vi "CalculateFit.vi"(8 "error in (no error)":errorcluster, 9 "Response in":dbl[][](array[numeric]), 10 "Stimulus in":dbl[][](array[numeric]), 11 "Head Impulse Fit in":refnum<class "Head Impulse Fit.lvclass">) -> (0 "error out":errorcluster, 3 "Head Impulse Fit out":refnum<class "Head Impulse Fit.lvclass">)   [LabVIEW 2016, in "Head Impulse Fit.lvclass"]
uses:
  Head Impulse Fit.lvclass
  Head Impulse Fit.lvclass/Head Impulse Fit.ctl
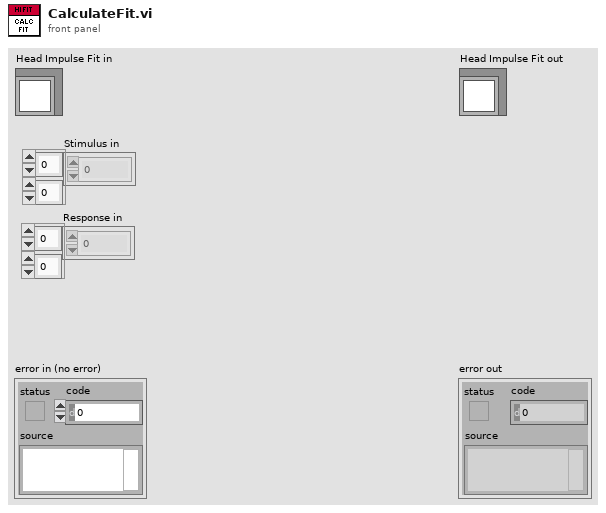
[diagram p1: front panel]
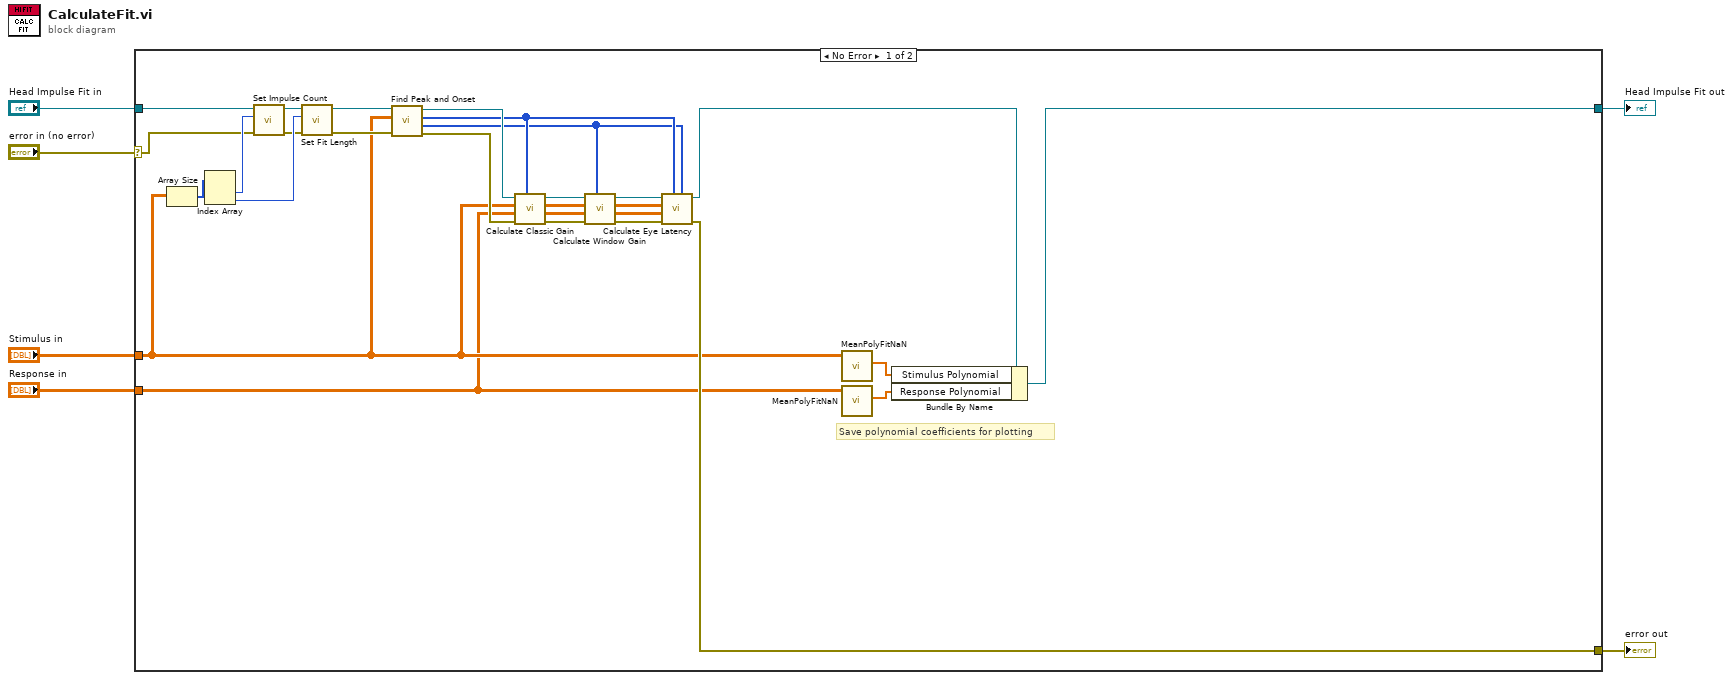
[diagram p0: block diagram]
diagram:
  n1 = case shown="No Error" "error in (no error)" {
    selector: "error in (no error)" -> [w29 w36]
    tunnel: [w16 w36] -> w5
    tunnel: [w9 w35] -> w3
    tunnel: "Head Impulse Fit in" -> [w32 w35]
    tunnel: "Stimulus in" -> [w12 _]
    tunnel: "Response in" -> [w11 _]
    frame No Error {
      # "Save polynomial coefficients for plotting"
      n2 = Array Size(array=w12) -> (size(s)=w34:i32[])
      n3 = Index Array(array=w34) -> (element #1=w31:i32, element #2=w30:i32)  [unwired: 2 in]
      n4 = call-dynamic "Set Impulse Count.vi"("error in (no error)"=w29, "Nr of Fit Impulses"=w31, "Abstract Fit in"=w32) -> ("error out"=w28:errorcluster, "Abstract Fit out"=w33:refnum<class "Head Impulse Fit.lvclass">)  [unwired: 7 in]
      n5 = call-dynamic "Set Fit Length.vi"("error in (no error)"=w28, "Length"=w30, "Abstract Fit in"=w33) -> ("error out"=w26:errorcluster, "Abstract Fit out"=w27:refnum<class "Head Impulse Fit.lvclass">)  [unwired: 7 in]
      n6 = call "Find Peak and Onset.vi"("error in (no error)"=w26, "Stimulus in"=w12, "Head Impulse Fit in"=w27) -> ("error out"=w24:errorcluster, "Onset Indicies"=w13:i32[], "Peak Indicies"=w14:i32[], "Head Impulse Fit out"=w25:refnum<class "Head Impulse Fit.lvclass">)  [unwired: 5 in]
      n7 = call "Calculate Classic Gain.vi"("Peak Indicies"=w14, "error in (no error)"=w24, "Response in"=w11, "Stimulus in"=w12, "Head Impulse Fit in"=w25) -> ("error out"=w21:errorcluster, "Response out"=w22:dbl[][], "Stimulus out"=w23:dbl[][], "Head Impulse Fit out"=w20:refnum<class "Head Impulse Fit.lvclass">)  [unwired: 3 in]
      n8 = call "Calculate Window Gain.vi"("Onset Indicies"=w13, "error in (no error)"=w21, "Response in"=w22, "Stimulus in"=w23, "Head Impulse Fit in"=w20) -> ("error out"=w17:errorcluster, "Response out"=w19:dbl[][], "Stimulus out"=w18:dbl[][], "Head Impulse Fit out"=w15:refnum<class "Head Impulse Fit.lvclass">)  [unwired: 3 in]
      n9 = call "Calculate Eye Latency.vi"("Onset Indicies"=w13, "Peak Indicies"=w14, "error in (no error)"=w17, "Response in"=w19, "Stimulus in"=w18, "Head Impulse Fit in"=w15) -> ("error out"=w16:errorcluster, "Head Impulse Fit out"=w10:refnum<class "Head Impulse Fit.lvclass">)  [unwired: 2 in, 2 out]
      n10 = call "MeanPolyFitNaN.vi"("Data"=w12) -> ("Polynomial Coefficients"=w7:dbl[])  [unwired: 9 in, 1 out]
      n11 = call "MeanPolyFitNaN.vi"("Data"=w11) -> ("Polynomial Coefficients"=w8:dbl[])  [unwired: 9 in, 1 out]
      n12 = Bundle By Name(cluster=w10, "Stimulus Polynomial"=w7, "Response Polynomial"=w8) -> (w9:refnum<class "Head Impulse Fit.lvclass">)
    }
    frame Error {
    }
  }
  "error out" <- w5
  "Head Impulse Fit out" <- w3
